vi "Transmit_Time(SubVI).vi"(10 "Number":i32, 11 "분":i32) -> (0 "강제 변환(x)":i32)   [LabVIEW 2023]
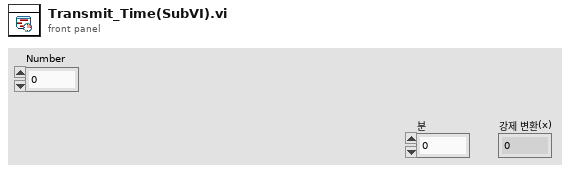
[diagram p1: front panel]
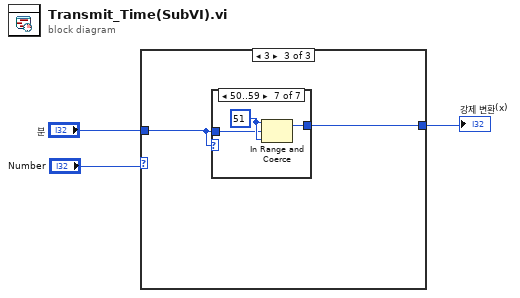
[diagram p0: block diagram]
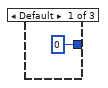
[diagram p2: hidden frame]
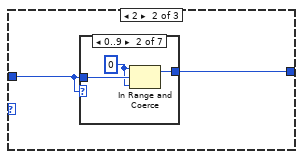
[diagram p3: hidden frame]
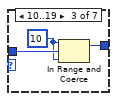
[diagram p5: hidden frame]
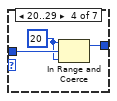
[diagram p6: hidden frame]
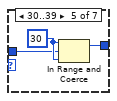
[diagram p7: hidden frame]
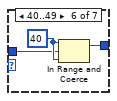
[diagram p8: hidden frame]
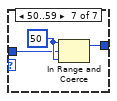
[diagram p9: hidden frame]
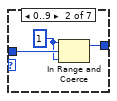
[diagram p11: hidden frame]
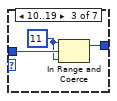
[diagram p12: hidden frame]
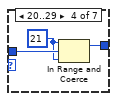
[diagram p13: hidden frame]
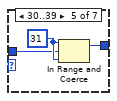
[diagram p14: hidden frame]
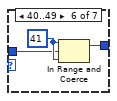
[diagram p15: hidden frame]
diagram:
  n1 = case shown="3" "Number" {
    tunnel: "분" -> [_ w6 w27]
    tunnel: [0 ("상위 리미트") w5 w26] -> w1
    frame Default {
    }
    frame 2 {
      n2 = case shown="0..9" w6 {
        tunnel: w6 -> [w7 w10 w13 w16 w18 w21 w24]
        tunnel: [w7 w9 w12 w15 w17 w20 w23] -> w5
        frame Default {
        }
        frame 0..9 {
          w8 = 0 ("상위 리미트")
          n3 = In Range and Coerce(upper limit=w8, x=w10, lower limit=w8) -> (coerced(x)=w9:i32)  [unwired: 1 out]
        }
        frame 10..19 {
          w11 = 10 ("상위 리미트")
          n4 = In Range and Coerce(upper limit=w11, x=w13, lower limit=w11) -> (coerced(x)=w12:i32)  [unwired: 1 out]
        }
        frame 20..29 {
          w14 = 20 ("상위 리미트")
          n5 = In Range and Coerce(upper limit=w14, x=w16, lower limit=w14) -> (coerced(x)=w15:i32)  [unwired: 1 out]
        }
        frame 30..39 {
          w19 = 30 ("상위 리미트")
          n6 = In Range and Coerce(upper limit=w19, x=w18, lower limit=w19) -> (coerced(x)=w17:i32)  [unwired: 1 out]
        }
        frame 40..49 {
          w22 = 40 ("상위 리미트")
          n7 = In Range and Coerce(upper limit=w22, x=w21, lower limit=w22) -> (coerced(x)=w20:i32)  [unwired: 1 out]
        }
        frame 50..59 {
          w25 = 50 ("상위 리미트")
          n8 = In Range and Coerce(upper limit=w25, x=w24, lower limit=w25) -> (coerced(x)=w23:i32)  [unwired: 1 out]
        }
      }
    }
    frame 3 {
      n9 = case shown="50..59" w27 {
        tunnel: w27 -> [w28 w31 w34 w37 w39 w42 w45]
        tunnel: [w28 w30 w33 w36 w38 w41 w44] -> w26
        frame Default {
        }
        frame 0..9 {
          w29 = 1 ("상위 리미트")
          n10 = In Range and Coerce(upper limit=w29, x=w31, lower limit=w29) -> (coerced(x)=w30:i32)  [unwired: 1 out]
        }
        frame 10..19 {
          w32 = 11 ("상위 리미트")
          n11 = In Range and Coerce(upper limit=w32, x=w34, lower limit=w32) -> (coerced(x)=w33:i32)  [unwired: 1 out]
        }
        frame 20..29 {
          w35 = 21 ("상위 리미트")
          n12 = In Range and Coerce(upper limit=w35, x=w37, lower limit=w35) -> (coerced(x)=w36:i32)  [unwired: 1 out]
        }
        frame 30..39 {
          w40 = 31 ("상위 리미트")
          n13 = In Range and Coerce(upper limit=w40, x=w39, lower limit=w40) -> (coerced(x)=w38:i32)  [unwired: 1 out]
        }
        frame 40..49 {
          w43 = 41 ("상위 리미트")
          n14 = In Range and Coerce(upper limit=w43, x=w42, lower limit=w43) -> (coerced(x)=w41:i32)  [unwired: 1 out]
        }
        frame 50..59 {
          w46 = 51 ("상위 리미트")
          n15 = In Range and Coerce(upper limit=w46, x=w45, lower limit=w46) -> (coerced(x)=w44:i32)  [unwired: 1 out]
        }
      }
    }
  }
  "강제 변환(x)" <- w1
